vi "SHA256CyclesCounter.vi"() -> ()   [LabVIEW 2024]
uses:
  <vilib>/OPCUA/controls/NodeId.ctl
  <vilib>/OPCUA/NI OPC UA Client.lvlib
  <vilib>/OPCUA/client/Multiple Read UInt32.vi
panel:
  out "Counters per second":u32
  out "Counter":u32(graph)
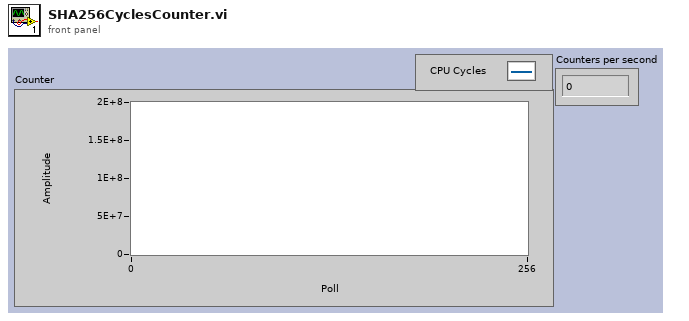
[diagram p1: front panel]
types:
  T1 = typedef "NodeId.ctl" = string
  T2 = typedef "OPC UA Client Refnum.ctl" = refnum<k21>
  T3 = typedef "OPC UA StatusCode.ctl" = u32
  T4 = cluster{"node ID":T1, "value ":u32, "timestamp":timestamp, "status":T3}[]
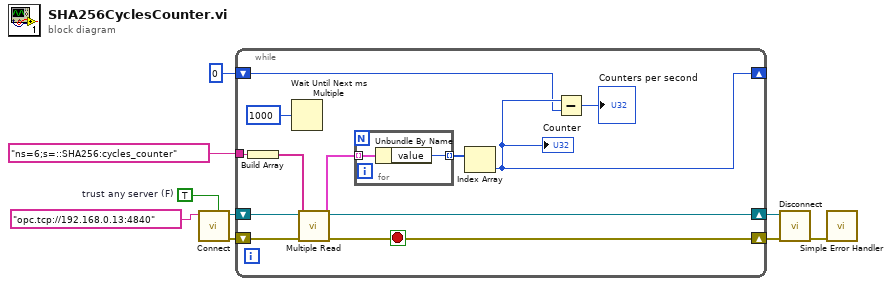
[diagram p0: block diagram]
diagram:
  w7 = TRUE  # trust any server (F)
  n1 = call <vilib>:"Connect.vi"("trust any server (F)"=w7, "server endpoint URL"="opc.tcp://192.168.0.13:4840") -> ("error out"=w4:errorcluster, "OPC UA client refnum out"=w6:T2)  [unwired: 7 in, 1 out]
  n2 = while {
    shift-right: [w20] -> w5
    shift-left: w6 -> [w18]
    shift-right: [w12] -> _
    shift-left: u32 0 ("Counter") -> [w11]
    shift-right: [w15] -> w3
    shift-left: w4 -> [w16]
    tunnel: T1 "ns=6;s=::SHA256:cycles_counter" ("node RU") -> [w14]
    stop <- w15 stop-if-true
    n3 = Build Array(w14) -> (w13:T1[])
    n4 = Wait Until Next ms Multiple(millisecond multiple=u32 1000) -> ()  [unwired: 1 out]
    n5 = call-poly <vilib>:"Multiple Read.vi"("error in (no error)"=w16, "node IDs"=w13, "OPC UA client refnum in"=w18) -> ("error out"=w15:errorcluster, "results"=w21:T4, "OPC UA client refnum out"=w20:T2)  [unwired: 5 in, 1 out]
    n6 = for {
      tunnel: w21 -> [w23] mode=indexing
      tunnel: [w22] -> w17 mode=indexing
      n7 = Unbundle By Name(w23) -> ("value"=w22:u32)
    }
    n8 = Index Array(array=w17) -> (element=w12:u32)  [unwired: 1 in]
    "Counter" <- w12
    n9 = Subtract(x=w12, y=w11) -> (x-y=→"Counters per second":u32)
  }
  n10 = call <vilib>:"Disconnect.vi"("error in (no error)"=w3, "OPC UA client refnum in"=w5) -> ("error out"=w9:errorcluster)  [unwired: 9 in]
  n11 = call <vilib>:"Simple Error Handler.vi"("error in (no error)"=w9) -> ()  [unwired: 4 in, 5 out]
